vi "TC_to_DSC.vi"(8 "error in (no error)":errorcluster, 10 "TC Cluster":T1) -> (0 "error out":errorcluster)   [LabVIEW 2013]
uses:
  Typedefs/TC-cluster.ctl
  <vilib>/Platform/browser.llb/Open URL in Default Browser (string).vi
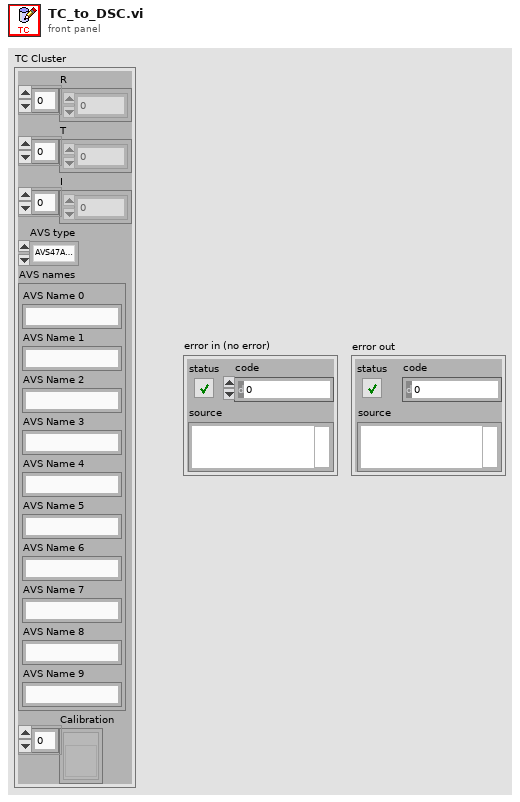
[diagram p1: front panel]
types:
  T1 = typedef "TC-cluster.ctl" = cluster{"R":dbl[], "T":dbl[], "I":dbl[], "AVS type":enum16{"AVS47A (GPIB interface)", "AVS47B (RS232 interface)", "AVS48", "AVS Emulation", "Impedance Bridge", "Disabled"}, "AVS names":cluster{"AVS Name 0":string, "AVS Name 1":string, "AVS Name 2":string, "AVS Name 3":string, "AVS Name 4":string, "AVS Name 5":string, "AVS Name 6":string, "AVS Name 7":string, "AVS Name 8":string, "AVS Name 9":string}, "Calibration":refnum<vi>[]}
  T2 = enum16{"AVS47A (GPIB interface)", "AVS47B (RS232 interface)", "AVS48", "AVS Emulation", "Impedance Bridge", "Disabled"}
  T3 = cluster{"AVS Name 0":string, "AVS Name 1":string, "AVS Name 2":string, "AVS Name 3":string, "AVS Name 4":string, "AVS Name 5":string, "AVS Name 6":string, "AVS Name 7":string, "AVS Name 8":string, "AVS Name 9":string}
  T4 = enum16{"CF", "CF_Z_Bridge", "MNK", "MNK_Z_Bridge"}
  T5 = cluster{"[0]":string, "[1]":string, "[2]":string, "[3]":string, "[4]":string, "[5]":string, "[6]":string, "[7]":string, "[8]":string, "[9]":string}
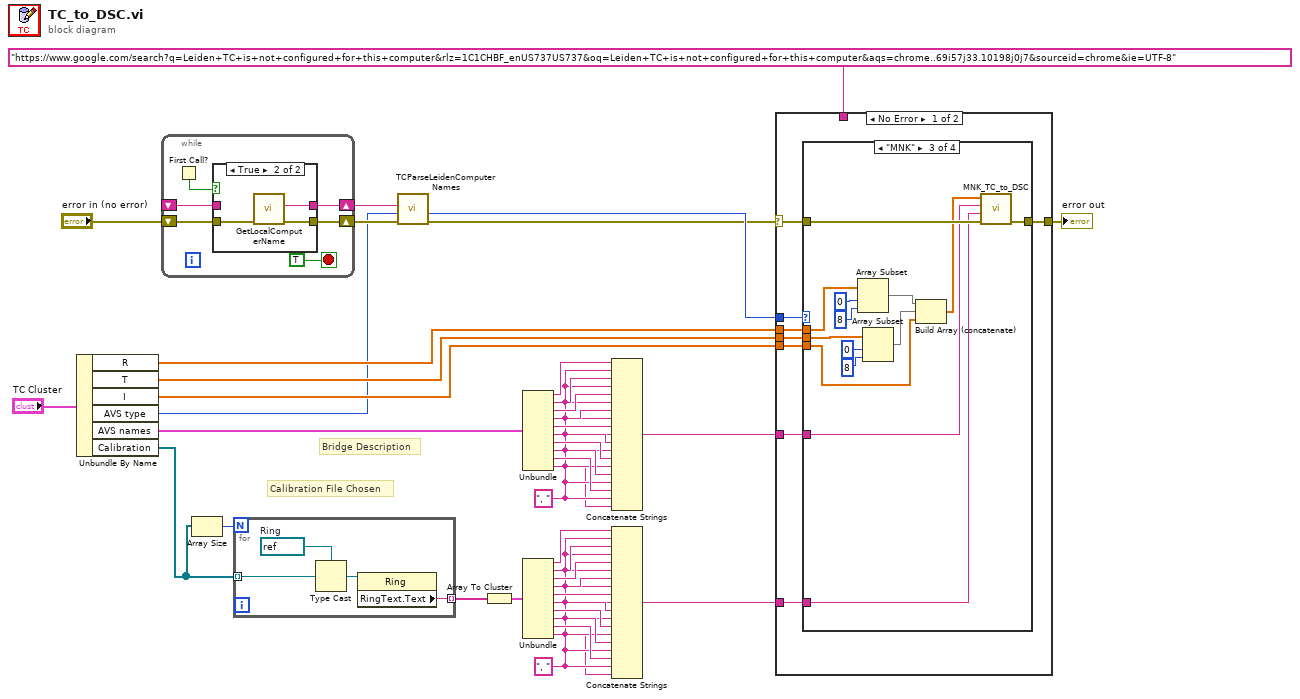
[diagram p0: block diagram]
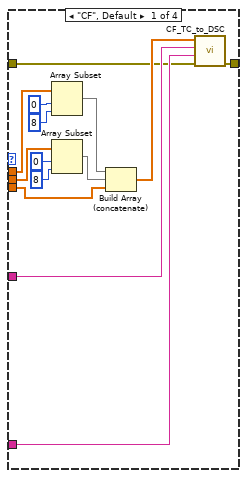
[diagram p3: hidden frame]
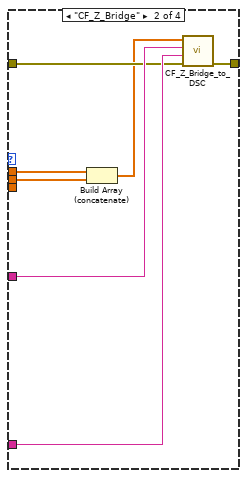
[diagram p4: hidden frame]
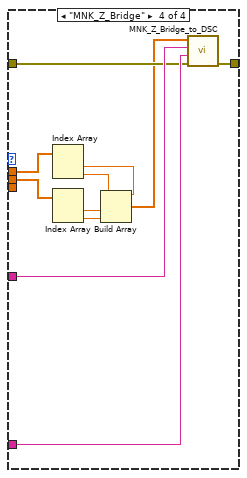
[diagram p5: hidden frame]
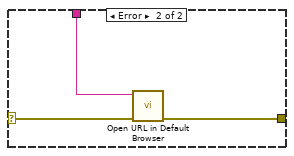
[diagram p6: hidden frame]
diagram:
  w18 = ", " ("string")
  w32 = ", " ("string")
  # "Bridge Description"
  # "Calibration File Chosen"
  n1 = Unbundle By Name("TC Cluster") -> ("R"=w8:dbl[], "T"=w7:dbl[], "I"=w6:dbl[], "AVS type"=w2:T2, "AVS names"=w5:T3, "Calibration"=w4:refnum<vi>[])
  n2 = while {
    shift-right: [w46] -> w12
    shift-left: "error in (no error)" -> [w43]
    shift-right: [w47] -> w1
    shift-left: _ -> [w42]
    stop <- TRUE stop-if-true
    n3 = First Call?() -> (First Call?: T/F=w45:bool)
    n4 = case shown="True" w45 {
      tunnel: [w49 w52] -> w47
      tunnel: [w48 w51] -> w46
      tunnel: w43 -> [w48 w50]
      tunnel: w42 -> [w49 _]
      frame False {
      }
      frame True {
        n5 = call "GetLocalComputerName.vi"("error in (no error)"=w50) -> ("error out"=w51:errorcluster, "Name"=w52:string)  [unwired: 8 in, 1 out]
      }
    }
  }
  n6 = Array Size(array=w4) -> (size(s)=w29:i32)
  n7 = for {
    N: w29 -> [_]
    tunnel: w4 -> [w56] mode=indexing
    tunnel: [w53] -> w28 mode=indexing
    w55 = refnum<vi> refnum  # Ring
    n8 = Type Cast(type=w55, x=w56) -> (*(type *) &x=w54:refnum<vi>)
    n9 = property class="Ring"(reference=w54) -> ("RingText.Text"=w53:string)  [unwired: 1 in, 2 out]
  }
  n10 = call "TCParseLeidenComputerNames.vi"("error in (no error)"=w12, "AVS type"=w2, "computer name"=w1) -> ("error out"=w13:errorcluster, "AVS Type"=w14:T4)  [unwired: 7 in]
  n11 = Array To Cluster(array=w28) -> (cluster=w16:T5)
  n12 = Unbundle(w5) -> ("AVS Name 0"=w41:string, "AVS Name 1"=w40:string, "AVS Name 2"=w39:string, "AVS Name 3"=w38:string, "AVS Name 4"=w37:string, "AVS Name 5"=w36:string, "AVS Name 6"=w35:string, "AVS Name 7"=w34:string, "AVS Name 8"=w33:string, "AVS Name 9"=w31:string)
  n13 = Unbundle(w16) -> ("[0]"=w27:string, "[1]"=w26:string, "[2]"=w25:string, "[3]"=w24:string, "[4]"=w23:string, "[5]"=w22:string, "[6]"=w21:string, "[7]"=w20:string, "[8]"=w19:string, "[9]"=w17:string)
  n14 = Concatenate Strings(w41, w32, w40, w32, w39, w32, w38, w32, w37, w32, w36, w32, w35, w32, w34, w32, w33, w32, w31) -> (w30:string)
  n15 = Concatenate Strings(w27, w18, w26, w18, w25, w18, w24, w18, w23, w18, w22, w18, w21, w18, w20, w18, w19, w18, w17) -> (w15:string)
  n16 = case shown="No Error" w13 {
    selector: w13 -> [w58 w113]
    tunnel: w30 -> [w64 _]
    tunnel: w15 -> [w63 _]
    tunnel: w14 -> [w62 _]
    tunnel: w8 -> [w61 _]
    tunnel: w7 -> [w60 _]
    tunnel: w6 -> [w59 _]
    tunnel: [w57 w112] -> w10
    tunnel: "https://www.google.com/search?q=Leiden+TC+is+not+configured+for+this+computer&rlz=1C1CHBF_enUS737US737&oq=Leiden+TC+is+not+configured+for+this+computer&aqs=chrome..69i57j33.10198j0j7&sourceid=chrome&ie=UTF-8" ("URL") -> [_ w111]
    frame No Error {
      n17 = case shown="\"MNK\"" w62 {
        tunnel: w61 -> [w67 w85 w98 w102]
        tunnel: w60 -> [w70 w84 w97 w101]
        tunnel: w59 -> [w71 _ w87 _]
        tunnel: w64 -> [w78 w83 w92 w106]
        tunnel: w63 -> [w77 w82 w93 w105]
        tunnel: w58 -> [w65 w81 w95 w104]
        tunnel: [w66 w80 w94 w103] -> w57
        frame "CF", Default {
          n18 = Array Subset(array=w67, index=0, length=8) -> (w69:dbl[])
          n19 = Array Subset(array=w70, index=0, length=8) -> (w68:dbl[])
          n20 = Build Array (concatenate)(w69, w68, w71) -> (w76:dbl[])
          n21 = call "CF_TC_to_DSC.vi"("error in (no error)"=w65, "calibration string"=w77, "description string"=w78, "dbl"=w76) -> ("error out"=w66:errorcluster)  [unwired: 7 in]
        }
        frame "CF_Z_Bridge" {
          n22 = Build Array (concatenate)(w85, w84) -> (w79:dbl[])
          n23 = call "CF_Z_Bridge_to_DSC.vi"("error in (no error)"=w81, "calibration string"=w82, "description string"=w83, "dbl"=w79) -> ("error out"=w80:errorcluster)  [unwired: 7 in]
        }
        frame "MNK" {
          n24 = Array Subset(array=w98, index=0, length=8) -> (w88:dbl[])
          n25 = Array Subset(array=w97, index=0, length=8) -> (w96:dbl[])
          n26 = Build Array (concatenate)(w88, w96, w87) -> (w86:dbl[])
          n27 = call "MNK_TC_to_DSC.vi"("error in (no error)"=w95, "calibration string"=w93, "description string"=w92, "dbl"=w86) -> ("error out"=w94:errorcluster)  [unwired: 7 in]
        }
        frame "MNK_Z_Bridge" {
          n28 = Index Array(array=w102) -> (element #1=w110:dbl, element #2=w109:dbl)  [unwired: 2 in]
          n29 = Index Array(array=w101) -> (element #1=w108:dbl, element #2=w107:dbl)  [unwired: 2 in]
          n30 = Build Array(w110, w109, w108, w107) -> (w100:dbl[])
          n31 = call "MNK_Z_Bridge_to_DSC.vi"("error in (no error)"=w104, "calibration string"=w105, "description string"=w106, "dbl"=w100) -> ("error out"=w103:errorcluster)  [unwired: 7 in]
        }
      }
    }
    frame Error {
      n32 = call-poly <vilib>:"Open URL in Default Browser.vi"("error in (no error)"=w113, "URL"=w111) -> ("error out"=w112:errorcluster)  [unwired: 4 in, 1 out]
    }
  }
  "error out" <- w10
